vi "deviceAnalysisTest_AnalogTach.vi"() -> ()   [LabVIEW 2017]
uses:
  <vilib>/addons/InsightCM/MessageBus/Base/controls/AlarmRuleEntry.ctl
  <vilib>/addons/InsightCM/Devices/Shared/DataAccessors/controls/channelType_StatusLookup.ctl
  <vilib>/addons/InsightCM/MessageBus/Base/KeyValuePairs.ctl
  <vilib>/addons/InsightCM/MessageBus/Base/ConfigurableMetric.ctl
  <vilib>/addons/InsightCM/Utilities/ChannelStatus/controls/status.ctl
  <vilib>/addons/InsightCM/Utilities/ChannelStatus/controls/statusState.ctl
  <vilib>/addons/InsightCM/Devices/Shared/ConfigurationParsing/controls/filePaths.ctl
panel:
  in  "Tab Control":T1(tab)
  in  "Root Directory":path=path "C:/Users/Administrator/Desktop/testDevice files/testIntegrationCutoff"
  in  "Configuration Files":T2={"AlarmRules"=path "AlarmRules.json", "MetricCfg"=path "MetricConfigs.json", "HierarchyNode"=path "Hierarchy.json", "DeviceModel"=path "DeviceModel.json"}
  in  "sampling info":cluster{"Fs":dbl, "#s":dbl}={"Fs"=10000.0, "#s"=10000.0} {"Fs" format="%.2p"}
  in  "Vibration":T3(array[cluster])
  in  "Tachometer":cluster{"RPM":sgl}={"RPM"=60.0} {"RPM" scale=1.0..6000.0}
  out "Waveform Graph":waveform(dbl)[](graph)
  out "Waveform Graph 2":waveform(sgl)[](graph)
  out "FeatureLookup":variant
  in  "stop":bool
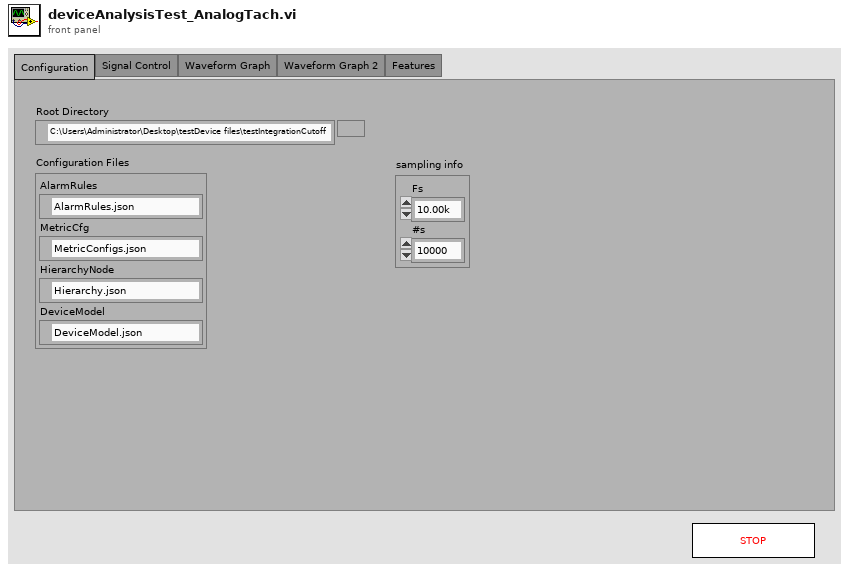
[diagram p1: front panel]
types:
  T1 = enum32{"Configuration", "Signal Control", "Waveform Graph", "Waveform Graph 2", "Features"}
  T2 = typedef "ConfigurationParsing.lvlib/filePaths.ctl" = cluster{"AlarmRules":path, "MetricCfg":path, "HierarchyNode":path, "DeviceModel":path}
  T3 = cluster{"order.":dbl, "mag (rms)":dbl, "phase (°)":dbl}[][]
  T4 = typedef "ChannelStatus.lvlib/statusState.ctl" = cluster{"channelAlias":string, "current":T5, "previous":T5, "changed":bool}
  T5 = typedef "ChannelStatus.lvlib/status.ctl" = enum16{"init", "ok", "open", "short", "outOfRange"}
  T6 = typedef "ConfigurableMetric.ctl" = cluster{"Id":i32, "MetricType":string, "Name":string, "Locked":bool, "Properties":T7}
  T7 = typedef "KeyValuePairs.ctl" = cluster{"Key":string, "Value":string}[]
  T8 = cluster{"order.":dbl, "mag (rms)":dbl, "phase (°)":dbl}[]
  T9 = typedef "AlarmRuleEntry.ctl" = cluster{"Id":i32, "State":string, "Path":string, "Message":string, "DeviceOnly":bool, "Configuration":cluster{"Condition":string, "SetPoint":string, "Type":string, "Hysteresis":dbl, "OnDelaySeconds":dbl, "OffDelaySeconds":dbl}, "Severity":i32}
  T10 = typedef "ConfigurationParsing.lvlib/DeviceConfigData.ctl" = cluster{"Device Info":T11, "AcquisitionProperties":variant, "Channels":variant[], "StreamingProperties":variant, "DeviceSystemProperties":variant}
  T11 = typedef "ConfigurationParsing.lvlib/deviceInfo.ctl" = cluster{"Config Version":string, "DeviceID":string}
  T12 = typedef "DeviceModel.ctl" = cluster{"AssetModel":T13, "SoftwareModel":T14}
  T13 = typedef "AssetModel.ctl" = cluster{"Id":i32, "PhysicalName":string, "LogicalName":string, "PluginCodename":string, "FirmwareInfo":string, "HardwareConfig":string, "SoftwareConfigId":i32, "HierarchyNodeId":i32}
  T14 = typedef "SoftwareModel.ctl" = cluster{"Id":i32, "DeviceAssetModelId":i32, "Version":string, "Config":string, "DeviceProperties":T7, "Channels":T15[]}
  T15 = typedef "BlueRidgeChannel.ctl" = cluster{"Id":i32, "ChannelId":string, "Name":string, "ChannelCategory":string, "ChannelType":string, "ChannelTypeList":string, "HierarchyNodeId":i32, "Enabled":bool, "Properties":T7, "MetricConfigurations":T16[]}
  T16 = typedef "MetricConfiguration.ctl" = cluster{"Id":i32, "ChannelCategory":string, "MeasurementType":string, "Metrics":T17[]}
  T17 = typedef "MetricInstance.ctl" = cluster{"Id":i32, "Codename":string, "DisplayName":string, "Unit":string, "PublishToHistorian":bool, "Unscaled":bool, "Locked":bool, "TagPath":string, "Properties":T7}
  T18 = cluster{"AlarmRules":variant, "MetricCfg":variant, "HierarchyNode":variant, "DeviceConfig":T10, "DeviceModel":T12}
  T19 = typedef "AnalysisDevice.ctl" = cluster{"Device Id":string, "Dynamic Channels":T20[], "Static Channels":T28[]}
  T20 = typedef "AnalysisDynamicChannel.ctl" = cluster{"ChannelName":string, "Sensor Type":T21, "Conversion Op":T22, "Features":T23[], "Data":waveform(sgl), "Speed":sgl, "SP Index":i32, "Properties":variant, "Data Valid":bool, "Calc Measurement Type":T27}
  T21 = typedef "AnalysisSensorType.ctl" = enum16{"Accelerometer", "Velocity", "Displacement", "Tachometer", "Tempertature ", "dynamicVoltage", "Voltage", "Current", "Microphone", "Resistance", "Digital Input", "<Unknown>"}
  T22 = typedef "AnalysisConversionOp.ctl" = enum16{"none", "singleInt", "doubleInt", "singleDiff", "doubleDiff"}
  T23 = typedef "AnalysisFeature.ctl" = cluster{"Type":i32, "Code Name":string, "Unit":string, "Display Name":string, "Value":sgl, "Start":dbl, "Stop":dbl, "Band Domain":T24, "Band Calc":T25, "Amplitude Scale":T26, "Tag Path":string}
  T24 = typedef "AnalysisBandDomain.ctl" = enum16{"Frequency", "CPM", "Orders"}
  T25 = typedef "AnalysisBandCalculation.ctl" = enum16{"Total", "Max", "Phase"}
  T26 = typedef "AnalysisBandAmplitudeScale.ctl" = enum16{"rms", "peak", "pk-pk", "phase", "<none>"}
  T27 = typedef "AnalysisCalculatedMeasurementType.ctl" = enum16{"acceleration", "velocity", "displacement", "tachometer", "speed", "temperature", "voltage", "current", "resistance", "digitalInput", "<Unknown>"}
  T28 = typedef "AnalysisStaticChannel.ctl" = cluster{"ChannelName":string, "Sensor Type":T21, "Features":T23[], "Properties":variant, "Data Valid":bool, "Calc Measurement Type":T27, "Acquisition Timestamp":timestamp}
  T29 = typedef "AnalysisState.ctl" = cluster{"Properties":cluster{"File Properties":variant, "Static Properties":variant, "Waveform Properties":variant}, "Properties Initialized?":bool, "Device":T19, "Speed Profiles":T30[]}
  T30 = typedef "AnalysisSpeedProfile.ctl" = cluster{"t0":dbl, "pulse positions":sgl[], "speed":dbl}
  T31 = typedef "AnalysisBOP.lvlib/AnalysisGroups.ctl" = cluster{"StaticChannels":T32[], "TachVibrationGroups":T34[]}
  T32 = typedef "AnalysisBOP.lvlib/GeneralStaticChanAnalysisCfg.ctl" = cluster{"Wfm Index":i32, "ChannelName":string, "ChannelID":string, "bounds":T33, "TagPath":string, "Triggerable":bool}
  T33 = typedef "ChannelStatus.lvlib/outOfRangeBounds.ctl" = cluster{"maximum":dbl, "minimum":dbl}
  T34 = typedef "AnalysisBOP.lvlib/TachVibrationGroupCfg.ctl" = cluster{"TachometerChanAnalysisConfig":T35, "AnalysisChannels":T36[]}
  T35 = typedef "AnalysisBOP.lvlib/TachometerChanAnalysisCfg.ctl" = cluster{"Wfm Index":i32, "ChannelName":string, "ChannelID":string, "PulsesPerRevolution":sgl, "TachometerThreshold":sgl, "TachometerSlope":string, "TachometerHysteresis":sgl, "sampleRate":dbl, "tachometerType":string, "Analysis Wfm Index":i32}
  T36 = typedef "AnalysisBOP.lvlib/VibrationChanAnalysisCfg.ctl" = cluster{"Wfm Index":i32, "ChannelName":string, "ChannelID":string, "speedRatio":dbl, "MeasurementType":string}
  T37 = typedef "channelType_StatusLookup.ctl" = enum16{"Static", "Dynamic"}
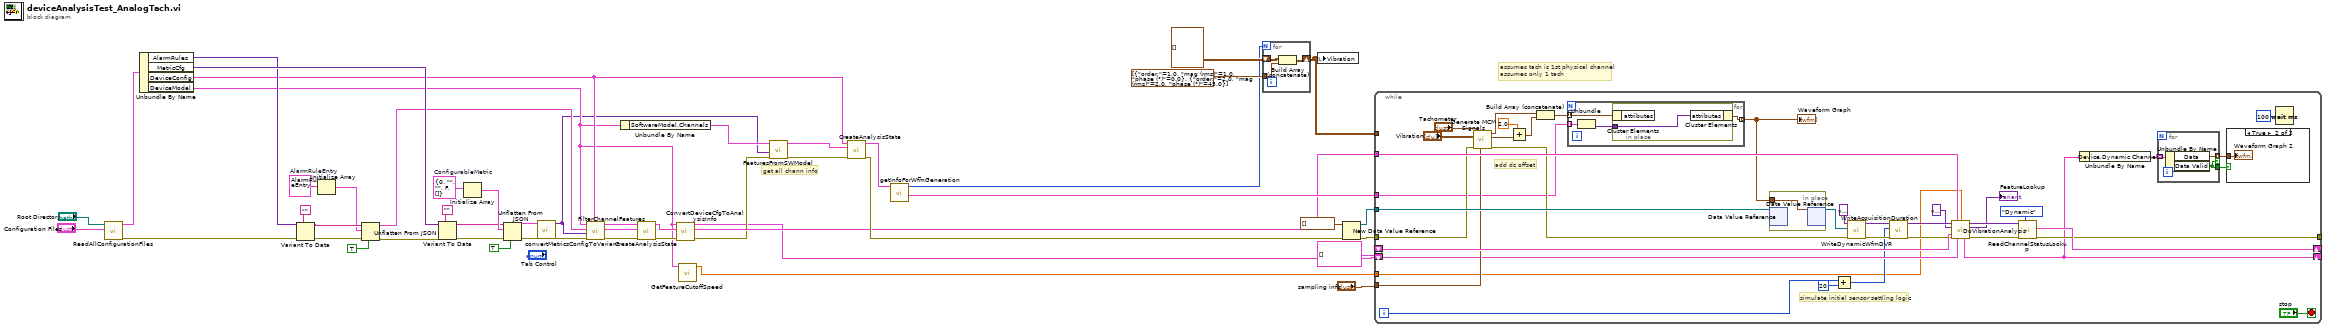
[diagram p0: block diagram]
diagram:
  w13 = T6 {"Id"=0, "MetricType"="", "Name"="", "Locked"=FALSE, "Properties"=[]}  # ConfigurableMetric
  w34 = T9 {"Id"=0, "State"="", "Path"="", "Message"="", "DeviceOnly"=FALSE, "Configuration"={"Condition"="", "SetPoint"="", "Type"="", "Hysteresis"=0.0, "OnDelaySeconds"=0.0, "OffDelaySeconds"=0.0}, "Severity"=0}  # AlarmRuleEntry
  # "assumes tach is 1st physical channel\nassumes only 1 tach"
  # "get all chann info"
  n1 = call <vilib>:"ReadAllConfigurationFiles.vi"("Configuration Files"="Configuration Files", "Root Directory"="Root Directory") -> ("error out"=w12:errorcluster, "Configuration"=w46:T18)  [unwired: 6 in, 2 out]
  n2 = Unbundle By Name(w46) -> ("AlarmRules"=w31:variant, "MetricCfg"=w40:variant, "DeviceConfig"=w16:T10, "DeviceModel"=w5:T12)
  n3 = Variant To Data(error in=w12, type="", Variant=w31) -> (data=w35:string, error out=w37:errorcluster)
  n4 = Initialize Array(w34) -> (w33:T9[])  [unwired: 1 in]
  n5 = Unflatten From JSON(JSON string=w35, type and defaults=w33, default null elements? (F)=TRUE, error in (no error)=w37) -> (value=w17:T9[], error out=w32:errorcluster)  [unwired: 3 in]
  n6 = Variant To Data(error in=w32, type="", Variant=w40) -> (data=w41:string, error out=w44:errorcluster)
  n7 = Initialize Array(w13) -> (w42:T6[])  [unwired: 1 in]
  n8 = Unflatten From JSON(JSON string=w41, type and defaults=w42, default null elements? (F)=TRUE, error in (no error)=w44) -> (value=w39:T6[], error out=w30:errorcluster)  [unwired: 3 in]
  n9 = call <vilib>:"convertMetricsConfigToVariant.vi"("error in (no error)"=w30, "MetricInstanceConfigs"=w39) -> ("error out"=w47:errorcluster, "metricInstanceConfig"=w2:variant)  [unwired: 8 in]
  n10 = call <vilib>:"FilterChannelFeatures.vi"("DeviceConfig"=w16, "error in (no error)"=w47, "Metric Lookup"=w2, "AlarmRules"=w17, "DeviceModel"=w5) -> ("error out"=w50:errorcluster, "Device"=w48:T19, "DeviceConfig Out"=w49:T10)  [unwired: 3 in, 1 out]
  n11 = Unbundle By Name(w5) -> ("SoftwareModel.Channels"=w14:T15[])
  n12 = call <vilib>:"CreateAnalysisState.vi"("error in (no error)"=w50, "Device"=w48, "DeviceConfig"=w49) -> ("error out"=w11:errorcluster, "Analysis State"=w8:T29)  [unwired: 7 in]
  n13 = call <vilib>:"ConvertDeviceCfgToAnalysisInfo.vi"("error in (no error)"=w11, "Analysis State"=w8, "DeviceModel"=w5) -> ("error out"=w9:errorcluster, "AnalysisGroups"=w10:T31, "Analysis State out"=w7:T29)  [unwired: 5 in, 1 out]
  n14 = call <vilib>:"GetFeatureCutoffSpeed.vi"("DeviceModel"=w5) -> ("featureCutoffSpeed"=w4:dbl)  [unwired: 10 in]
  n15 = call <vilib>:"FeaturesFromSWModel.vi"("error in (no error)"=w9, "Band Cache"=w2, "Channels"=w14) -> ("error out"=w3:errorcluster, "Device"=w1:T19)  [unwired: 7 in]
  n16 = call <vilib>:"CreateAnalysisState.vi"("error in (no error)"=w3, "Device"=w1, "DeviceConfig"=w16) -> ("error out"=w15:errorcluster, "Analysis State"=w18:T29)  [unwired: 7 in]
  n17 = call <vilib>:"_getInfoForWfmGeneration.vi"("Analysis State"=w18) -> ("wfm info"=w19:cluster{i32, "variant":variant}[], "number of channels"=w20:i32)  [unwired: 9 in]
  n18 = for {
    N: w20 -> [_]
    tunnel: T8 [{"order."=1.0, "mag (rms)"=1.0, "phase (°)"=0.0}, {"order."=2.0, "mag (rms)"=2.0, "phase (°)"=45.0}] ("Vibration") -> [w53]
    shift-right: [w52] -> w22
    shift-left: T3 [] -> [w51]
    n19 = Build Array (concatenate)(w51, w53) -> (w52:T3)
  }
  n20 = local write "Vibration"(w22) -> ()
  n21 = New Data Value Reference(data value=waveform(sgl)[] [] ("wfmData"), error in=w15) -> (data value reference=w26:refnum<data-value>, error out=w27:errorcluster)
  n22 = while {
    tunnel: w27 -> [w80]
    tunnel: w10 -> [w92]
    shift-right: [w91] -> _
    shift-left: T4[] [] ("channel status") -> [w90]
    tunnel: w26 -> [w85]
    tunnel: "sampling info" -> [w77]
    tunnel: w22 -> [_]
    tunnel: [w71] -> _
    tunnel: w19 -> [w70]
    shift-right: [w67] -> _
    shift-left: w7 -> [w68]
    tunnel: w4 -> [w54]
    i -> [w61]
    stop <- "stop" stop-if-true
    # "add dc offset"
    # "simulate initial sensor settling logic"
    n23 = call <vilib>:"Generate MCM Signals.vi"("sampling info"=w77, "error in"=w80, "Vibration"="Vibration", "Tachometer"="Tachometer") -> ("error out"=w79:errorcluster, "Vibration signals"=w57:waveform(dbl)[], "Tach signal"=w62:waveform(dbl))  [unwired: 5 in]
    n24 = Add(x=2.0, y=w57) -> (x+y=w56:waveform(dbl)[])
    n25 = Build Array (concatenate)(w62, w56) -> (w63:waveform(dbl)[])
    n26 = for {
      tunnel: w63 -> [w99] mode=indexing
      tunnel: w70 -> [w100] mode=indexing
      tunnel: [w98] -> w69 mode=indexing
      n27 = Unbundle(w100) -> ("variant"=w97:variant)  [unwired: 1 out]
      n28 = in-place {
        in-place-border: w97 -> [w101]
        n29 = in-place-cluster #1(w99) -> ()  [unwired: 1 out]
        n30 = in-place-cluster #1("attributes"=w101) -> (w98:waveform(dbl))
      }
    }
    "Waveform Graph" <- w69
    n31 = in-place {
      in-place-border: w69 -> [w102]
      n32 = in-place-dvr #2(w85) -> ()  [unwired: 2 out]
      n33 = in-place-dvr #2(w102) -> (w84:refnum<data-value>)  [unwired: 1 out]
    }
    n34 = Add(x=w61, y=20) -> (x+y=w60:i32)
    n35 = call <vilib>:"WriteDynamicWfmDVR.vi"("error in (no error)"=w79, "dynamic Wfm DVR"=w84, "variant"=variant) -> ("error out"=w89:errorcluster, "variant"=w88:variant)  [unwired: 7 in]
    n36 = call <vilib>:"WriteAcquisitionDuration.vi"("error in (no error)"=w89, "acquisitionDuration"=w60, "variant"=w88) -> ("error out"=w86:errorcluster, "variant"=w87:variant)  [unwired: 7 in]
    n37 = call <vilib>:"DoVibrationAnalysis.vi"("variant"=w87, "AnalysisGroups"=w92, "FeatureSpeedCutoff"=w54, "featureLookup"=variant, "channel status"=w90, "error in (no error)"=w86, "Analysis State"=w68) -> ("variant out"=w74:variant, "FeatureLookup"=→"FeatureLookup":variant, "Analysis State Out"=w67:T29, "error out"=w73:errorcluster)  [unwired: 4 in, 1 out]
    n38 = call <vilib>:"ReadChannelStatusLookup.vi"("channel type"=channelType_StatusLookup."Dynamic", "error in (no error)"=w73, "variant"=w74) -> ("error out"=w71:errorcluster, "channel status"=w91:T4[])  [unwired: 6 in, 1 out]
    n39 = Unbundle By Name(w67) -> ("Device.Dynamic Channels"=w66:T20[])
    n40 = for {
      tunnel: w66 -> [w96] mode=indexing
      tunnel: [w95] -> w65 mode=indexing if=w94
      tunnel: [w94] -> w58
      n41 = Unbundle By Name(w96) -> ("Data"=w95:waveform(sgl), "Data Valid"=w94:bool)
    }
    n42 = case shown="True" w58 {
      tunnel: w65 -> [_ w93]
      frame False {
      }
      frame True {
        "Waveform Graph 2" <- w93
      }
    }
    n43 = Wait (ms)(milliseconds to wait=u32 100) -> ()  [unwired: 1 out]
  }
